vi "Initialize_WithSerialCommunication.vi"(8 "error in":errorcluster, 11 "Comport":refnum<visa-resource-name>="COM20") -> (0 "error out":errorcluster, 3 "Transport Parameters":T1={"Serial Communication"={"Comport"="", "Transporter File Path"=path "", "No Response Timeout Ms"=10000, "Response Complete Timeout Ms"=10000, "Max Rx Length"=10000, "Baud Rate"=20}, "Selected Transport"=enum."Serial Communication Port", "Selected Transporter File Path"=path ""} {"Serial Communication"."Baud Rate" items=["75"=75, "110"=110, "134"=134, "150"=150, "300"=300, "600"=600, "1200"=1200, "1800"=1800, "2400"=2400, "4800"=4800, "7200"=7200, "9600"=9600, "14400"=14400, "19200"=19200, "28800"=28800, "38400"=38400, "56000"=56000, "57600"=57600, "115200"=115200, "128000"=128000, "230400"=230400]})   [LabVIEW 2020]
doc: "Initializes the library with a serial comport as the transport method"
uses:
  Controls/ConnectionParameters.ctl
  Controls/SupportedTransports.ctl
panel:
  out "FirmataFirmwareVersion":string="v2.5"
  out "FirmataFirmwareName":string="StandardFirmata.ino"
  in  "Baud Rate":u32(ring)=57600 items=["75"=75, "110"=110, "134"=134, "150"=150, "300"=300, "600"=600, "1200"=1200, "1800"=1800, "2400"=2400, "4800"=4800, "7200"=7200, "9600"=9600, "14400"=14400, "19200"=19200, "28800"=28800, "38400"=38400, "56000"=56000, "57600"=57600, "115200"=115200, "128000"=128000, "230400"=230400]
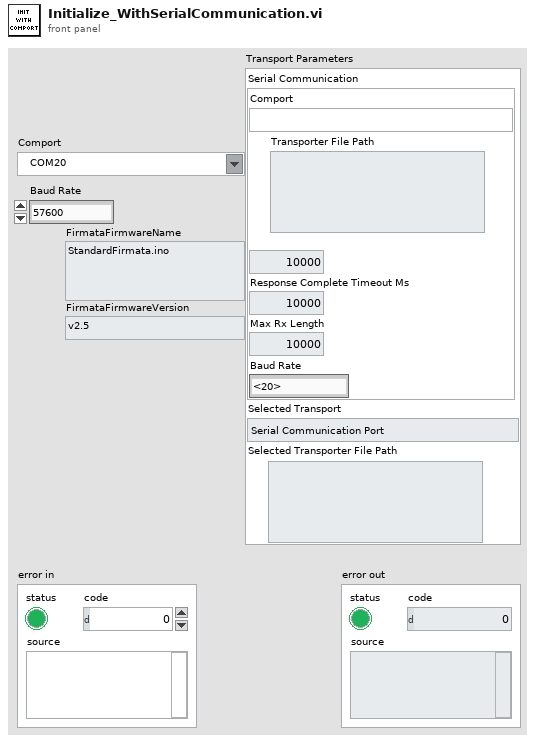
[diagram p1: front panel]
types:
  T1 = typedef "ConnectionParameters.ctl" = cluster{"Serial Communication":cluster{"Comport":refnum<visa-resource-name>, "Transporter File Path":path, "No Response Timeout Ms":u32, "Response Complete Timeout Ms":u32, "Max Rx Length":u32, "Baud Rate":u32}, "Selected Transport":T2, "Selected Transporter File Path":path}
  T2 = typedef "SupportedTransports.ctl" = enum16{"Serial Communication Port"}
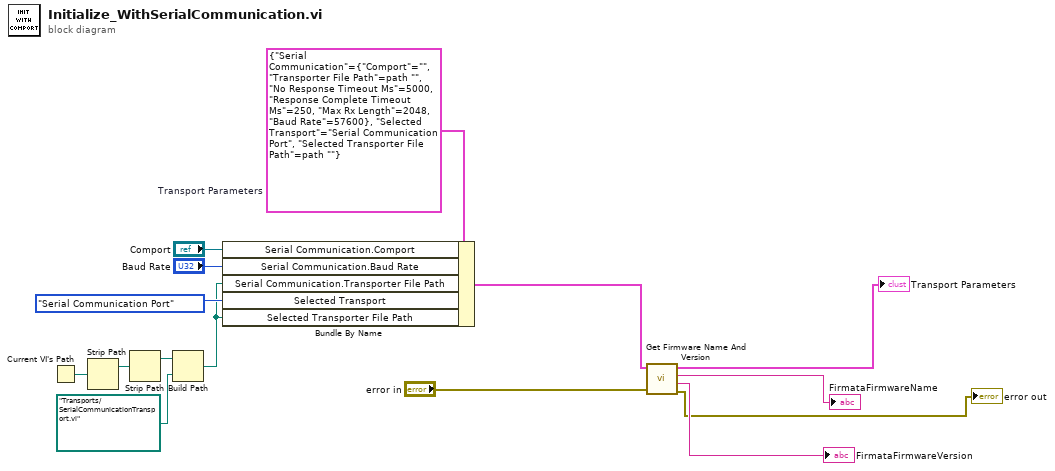
[diagram p0: block diagram]
diagram:
  w14 = T1 {"Serial Communication"={"Comport"="", "Transporter File Path"=path "", "No Response Timeout Ms"=5000, "Response Complete Timeout Ms"=250, "Max Rx Length"=2048, "Baud Rate"=57600}, "Selected Transport"=enum."Serial Communication Port", "Selected Transporter File Path"=path ""}  # Transport Parameters
  n1 = Current VI's Path() -> (path=w9:path)
  n2 = Strip Path(path=w9) -> (stripped path=w8:path)  [unwired: 1 out]
  n3 = Strip Path(path=w8) -> (stripped path=w7:path)  [unwired: 1 out]
  n4 = Build Path(base path=w7, name or relative path=path "Transports/SerialCommunicationTransport.vi" ("Serial Communication.Transporter File Path")) -> (appended path=w5:path)
  n5 = Bundle By Name(cluster=w14, "Serial Communication.Comport"="Comport", "Serial Communication.Baud Rate"="Baud Rate", "Serial Communication.Transporter File Path"=w5, "Selected Transport"=SupportedTransports."Serial Communication Port", "Selected Transporter File Path"=w5) -> (w12:T1)
  n6 = call "Get Firmware Name And Version.vi"("error in (no error)"="error in", "Transport Parameters in"=w12) -> ("error out"=→"error out":errorcluster, "FirmataFirmwareVersion"=→"FirmataFirmwareVersion":string, "FirmataFirmwareName"=→"FirmataFirmwareName":string, "Transport Parameters out"=→"Transport Parameters":T1)  [unwired: 6 in]
